vi "onHttpHead.vi"(8 "error in":errorcluster, 10 "httpRequest":refnum<class "httpRequest.lvclass">, 11 "http-client in":refnum<class "HttpClient.Basic.lvclass">) -> (0 "error out":errorcluster, 2 "httpResponse":refnum<class "httpResponse.lvclass">, 3 "http-client out":refnum<class "HttpClient.Basic.lvclass">)   [LabVIEW 2020, in "httpClient.lvlib" / "HttpClient.Basic.lvclass"]
uses:
  HttpClient.Basic.lvclass
  HttpClient.Basic.lvclass/HttpClient.Basic.ctl
  <vilib>/httpClient/LabVIEWHTTPClient.lvlib
  httpRequest/httpRequest.lvclass
  httpResponse/httpResponse.lvclass
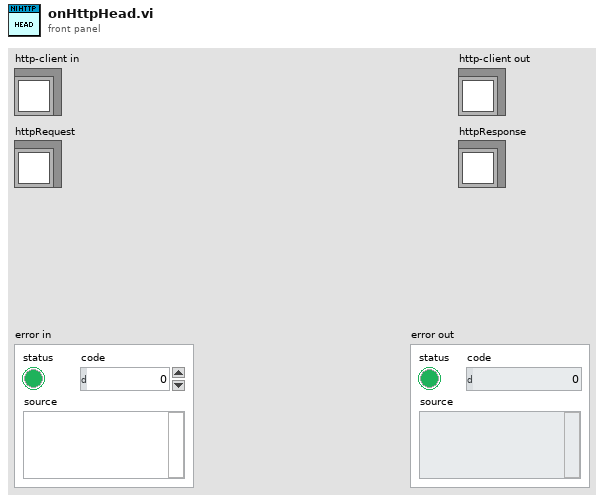
[diagram p1: front panel]
types:
  T1 = typedef "LabVIEWHTTPClient.lvlib/ClientHandle.ctl" = refnum<k1>
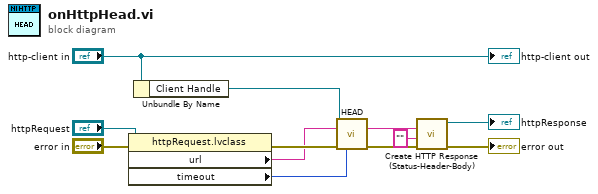
[diagram p0: block diagram]
diagram:
  n1 = property class="httpRequest.lvclass"(reference="httpRequest", error in="error in") -> (error out=w8:errorcluster, "url"=w7:string, "timeout"=w6:i32)  [unwired: 1 out]
  n2 = Unbundle By Name("http-client in") -> ("Client Handle"=w11:T1)
  n3 = call <vilib>:"HEAD.vi"("client handle"=w11, "url"=w7, "error in (no error)"=w8, "timeout (10000)"=w6) -> ("headers"=w2:string, "error out"=w5:errorcluster)  [unwired: 9 in, 1 out]
  n4 = call "Create HTTP Response (Status-Header-Body).vi"("error in"=w5, "body"="", "Headers w/ status line(s)"=w2) -> ("error out"=→"error out":errorcluster, "httpResponse out"=→"httpResponse":refnum<class "httpResponse.lvclass">)  [unwired: 7 in]
  "http-client out" <- "http-client in"
